vi "ReadForLoop.vi"(1 "reference":refnum<vi>) -> (0 "ForLoop":T6)   [LabVIEW 2013]
uses:
  <vilib>/Utility/miscctls.llb/LVBoundsTypeDef.ctl
  <vilib>/Utility/miscctls.llb/LVPositionTypeDef.ctl
  <vilib>/Utility/miscctls.llb/LVRectTypeDef.ctl
  <vilib>/Utility/miscctls.llb/LVBreakpointStatusEnum.ctl
  <vilib>/Utility/miscctls.llb/LVParallelSchedulesEnum.ctl
panel:
  out "error out 41":errorcluster
  out "error out 40":errorcluster
  out "error out 39":errorcluster
  out "error out 38":errorcluster
  out "error out 37":errorcluster
  out "error out 36":errorcluster
  out "error out 35":errorcluster
  out "error out 34":errorcluster
  out "error out 33":errorcluster
  out "error out 32":errorcluster
  out "error out 31":errorcluster
  out "error out 30":errorcluster
  out "error out 29":errorcluster
  out "error out 28":errorcluster
  out "error out 27":errorcluster
  out "error out 26":errorcluster
  out "error out 25":errorcluster
  out "error out 24":errorcluster
  out "error out 23":errorcluster
  out "error out 22":errorcluster
  out "error out 21":errorcluster
  out "error out 20":errorcluster
  out "error out 19":errorcluster
  out "error out 18":errorcluster
  out "error out 17":errorcluster
  out "error out 16":errorcluster
  out "error out 15":errorcluster
  out "error out 14":errorcluster
  out "error out 13":errorcluster
  out "error out 12":errorcluster
  out "error out 11":errorcluster
  out "error out 10":errorcluster
  out "error out 9":errorcluster
  out "error out 8":errorcluster
  out "error out 7":errorcluster
  out "error out 6":errorcluster
  out "error out 5":errorcluster
  out "error out 4":errorcluster
  out "error out 3":errorcluster
  out "error out 2":errorcluster
  out "error out":errorcluster
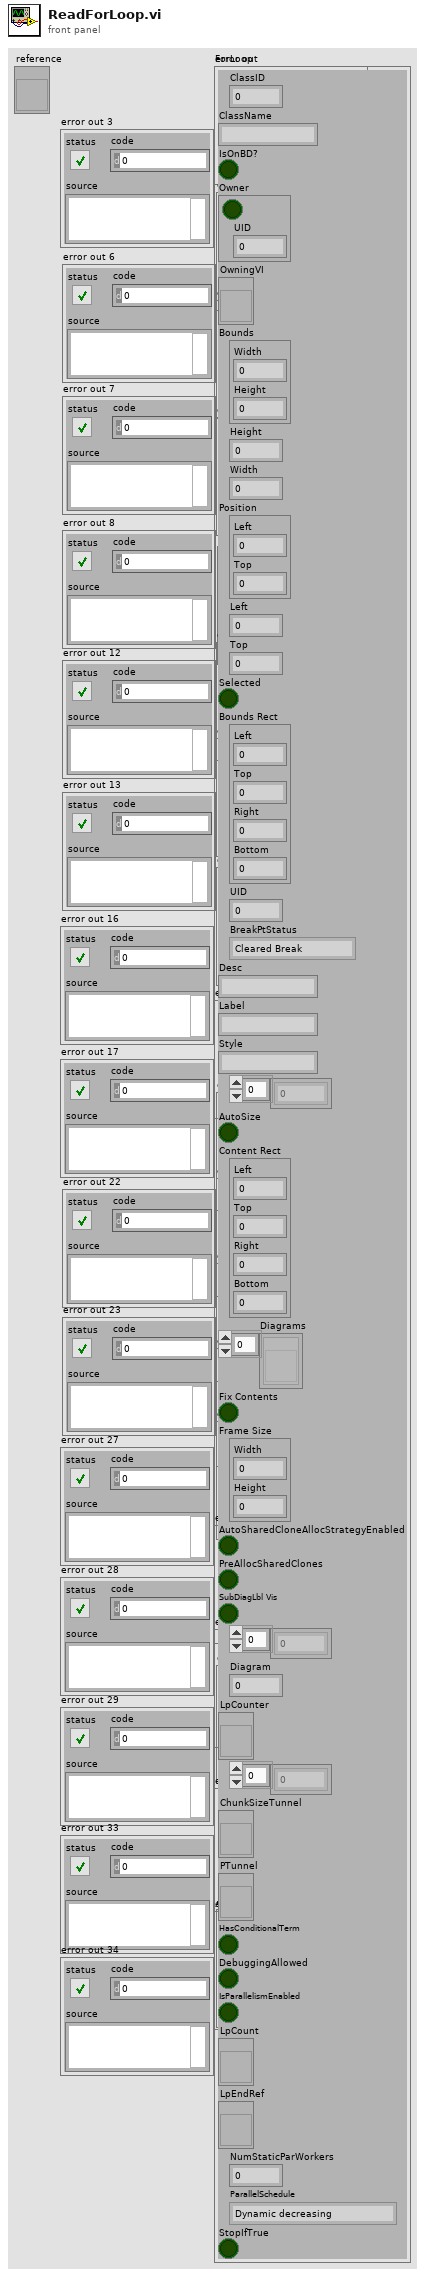
[diagram p1: front panel]
types:
  T1 = typedef "LVBoundsTypeDef.ctl" = cluster{"Width":u32, "Height":u32}
  T2 = typedef "LVPositionTypeDef.ctl" = cluster{"Left":i32, "Top":i32}
  T3 = typedef "LVRectTypeDef.ctl" = cluster{"Left":i16, "Top":i16, "Right":i16, "Bottom":i16}
  T4 = typedef "LVBreakpointStatusEnum.ctl" = enum8{"Cleared Break", "Enabled Break", "Disabled Break"}
  T5 = typedef "LVParallelSchedulesEnum.ctl" = enum8{"Dynamic decreasing", "Dynamic fixed size", "Static block", "Static block-cyclic"}
  T6 = cluster{"ClassID":u32, "ClassName":string, "IsOnBD?":bool, "Owner":cluster{bool, "UID":i32}, "OwningVI":refnum<vi>, "Bounds":T1, "Height":u32, "Width":u32, "Position":T2, "Left":i32, "Top":i32, "Selected":bool, "Bounds Rect":T3, "UID":i32, "BreakPtStatus":T4, "Desc":string, "Label":string, "Style":string, "Terms[]":i32[], "AutoSize":bool, "Content Rect":T3, "Diagrams":refnum<vi>[], "Fix Contents":bool, "Frame Size":T1, "AutoSharedCloneAllocStrategyEnabled":bool, "PreAllocSharedClones":bool, "SubDiagLbl Vis":bool, "Tunnels[]":i32[], "Diagram":i32, "LpCounter":refnum<vi>, "ShiftRegs[]":i32[], "ChunkSizeTunnel":refnum<vi>, "PTunnel":refnum<vi>, "HasConditionalTerm":bool, "DebuggingAllowed":bool, "IsParallelismEnabled":bool, "LpCount":refnum<vi>, "LpEndRef":refnum<vi>, "NumStaticParWorkers":i32, "ParallelSchedule":T5, "StopIfTrue":bool}
  T7 = cluster{"ClassID":u32, "ClassName":string, "IsOnBD?":bool, "Cluster":cluster{bool, "UID":i32}, "OwningVI":refnum<vi>, "Bounds":T1, "Height":u32, "Width":u32, "Position":T2, "Left":i32, "Top":i32, "Selected":bool, "Bounds Rect":T3, "UID":i32, "BreakPtStatus":T4, "Desc":string, "Text":string, "Style":string, i32[], "AutoSize":bool, "Content Rect":T3, "Diagrams":refnum<vi>[], "Fix Contents":bool, "Frame Size":T1, "AutoSharedCloneAllocStrategyEnabled":bool, "PreAllocSharedClones":bool, "SubDiagLbl Vis":bool, i32[], "UID":i32, "LpCounter":refnum<vi>, i32[], "ChunkSizeTunnel":refnum<vi>, "PTunnel":refnum<vi>, "HasConditionalTerm":bool, "DebuggingAllowed":bool, "IsParallelismEnabled":bool, "LpCount":refnum<vi>, "LpEndRef":refnum<vi>, "NumStaticParWorkers":i32, "ParallelSchedule":T5, "StopIfTrue":bool}
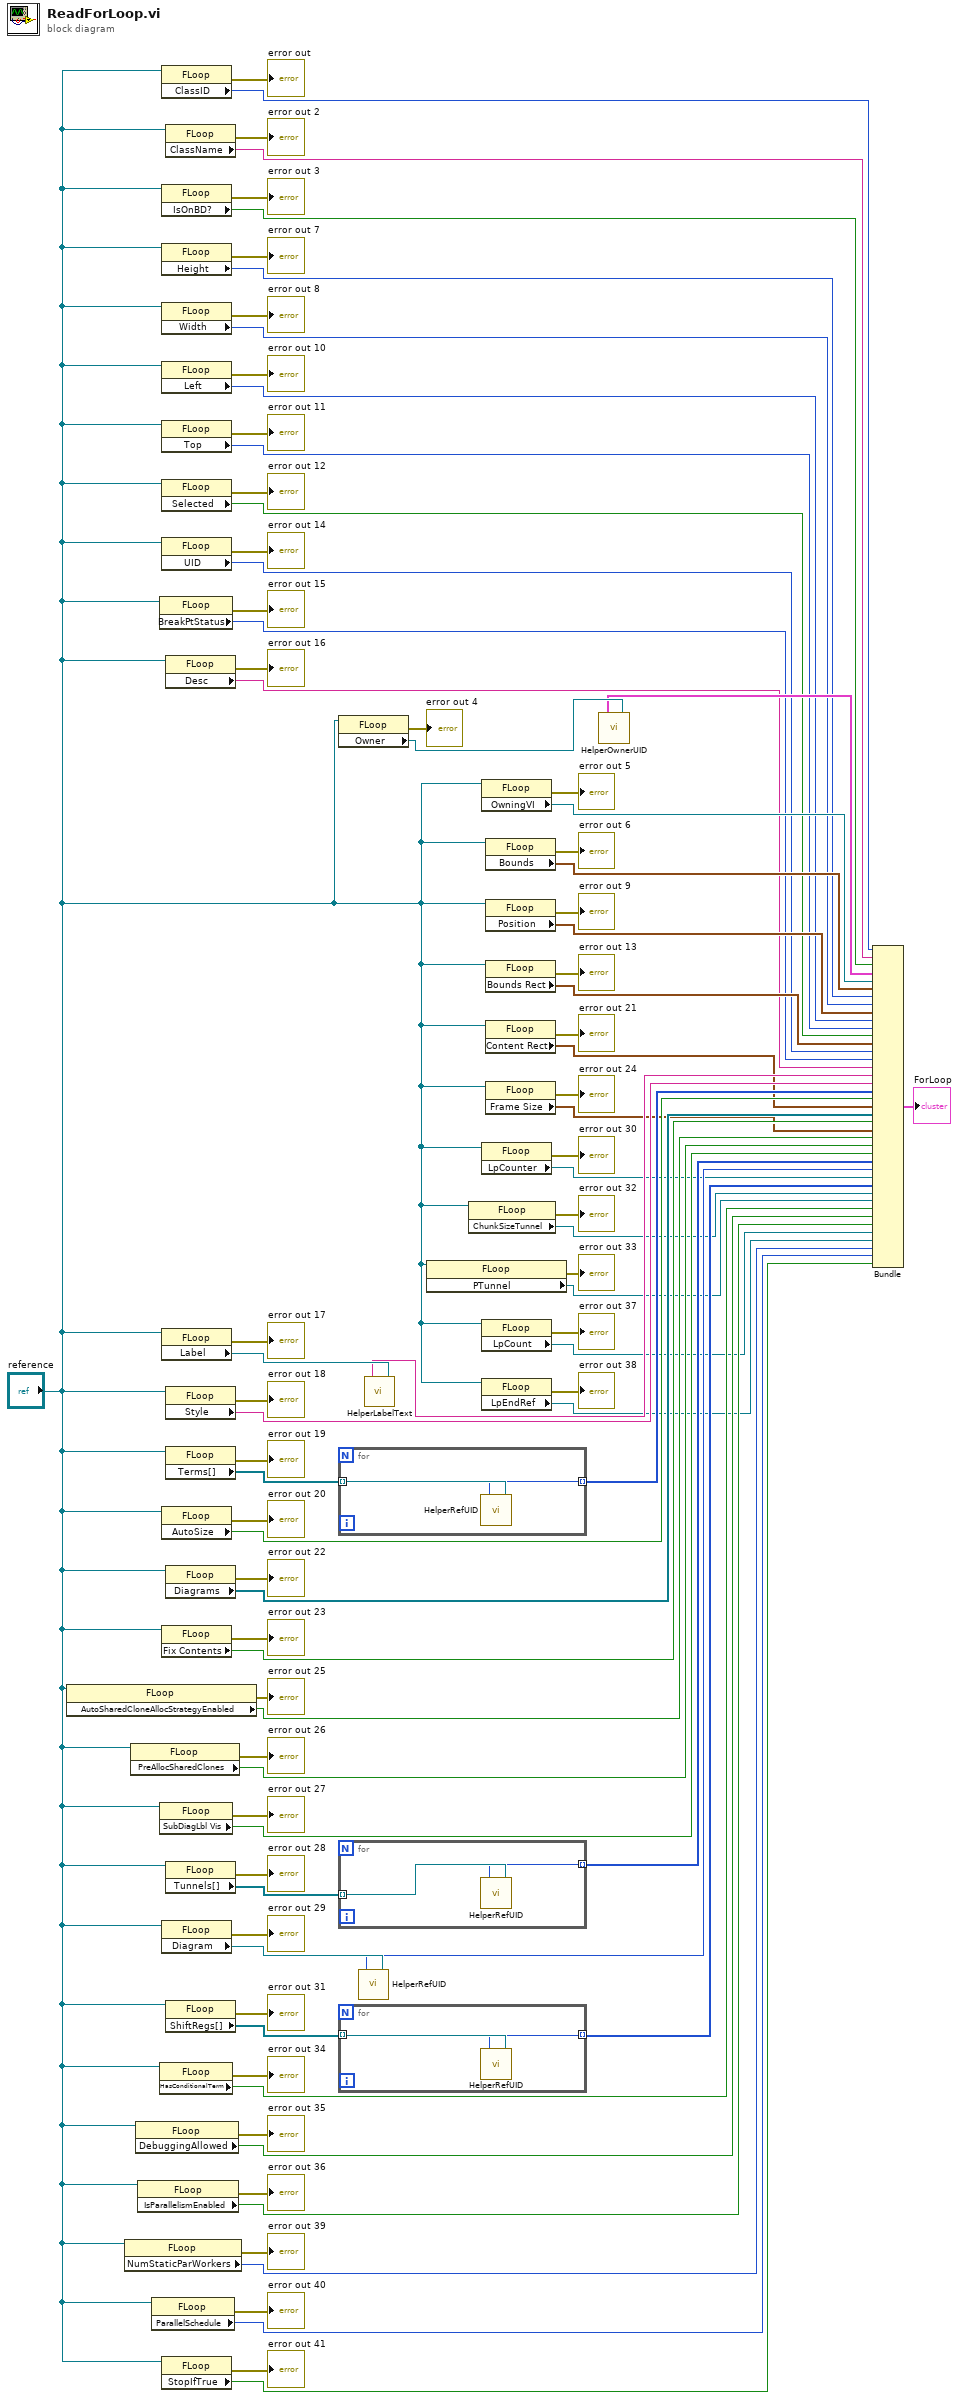
[diagram p0: block diagram]
diagram:
  n1 = property class="FLoop"(reference="reference") -> (error out=→"error out 25":errorcluster, "AutoSharedCloneAllocStrategyEnabled"=w37:bool)  [unwired: 1 in, 1 out]
  n2 = property class="FLoop"(reference="reference") -> (error out=→"error out 39":errorcluster, "NumStaticParWorkers"=w6:i32)  [unwired: 1 in, 1 out]
  n3 = property class="FLoop"(reference="reference") -> (error out=→"error out 26":errorcluster, "PreAllocSharedClones"=w35:bool)  [unwired: 1 in, 1 out]
  n4 = property class="FLoop"(reference="reference") -> (error out=→"error out 35":errorcluster, "DebuggingAllowed"=w14:bool)  [unwired: 1 in, 1 out]
  n5 = property class="FLoop"(reference="reference") -> (error out=→"error out 36":errorcluster, "IsParallelismEnabled"=w12:bool)  [unwired: 1 in, 1 out]
  n6 = property class="FLoop"(reference="reference") -> (error out=→"error out 40":errorcluster, "ParallelSchedule"=w4:T5)  [unwired: 1 in, 1 out]
  n7 = property class="FLoop"(reference="reference") -> (error out=→"error out 15":errorcluster, "BreakPtStatus"=w59:T4)  [unwired: 1 in, 1 out]
  n8 = property class="FLoop"(reference="reference") -> (error out=→"error out 27":errorcluster, "SubDiagLbl Vis"=w33:bool)  [unwired: 1 in, 1 out]
  n9 = property class="FLoop"(reference="reference") -> (error out=→"error out 34":errorcluster, "HasConditionalTerm"=w16:bool)  [unwired: 1 in, 1 out]
  n10 = property class="FLoop"(reference="reference") -> (error out=→"error out":errorcluster, "ClassID"=w88:u32)  [unwired: 1 in, 1 out]
  n11 = property class="FLoop"(reference="reference") -> (error out=→"error out 3":errorcluster, "IsOnBD?"=w84:bool)  [unwired: 1 in, 1 out]
  n12 = property class="FLoop"(reference="reference") -> (error out=→"error out 7":errorcluster, "Height"=w75:u32)  [unwired: 1 in, 1 out]
  n13 = property class="FLoop"(reference="reference") -> (error out=→"error out 8":errorcluster, "Width"=w73:u32)  [unwired: 1 in, 1 out]
  n14 = property class="FLoop"(reference="reference") -> (error out=→"error out 10":errorcluster, "Left"=w69:i32)  [unwired: 1 in, 1 out]
  n15 = property class="FLoop"(reference="reference") -> (error out=→"error out 11":errorcluster, "Top"=w67:i32)  [unwired: 1 in, 1 out]
  n16 = property class="FLoop"(reference="reference") -> (error out=→"error out 12":errorcluster, "Selected"=w65:bool)  [unwired: 1 in, 1 out]
  n17 = property class="FLoop"(reference="reference") -> (error out=→"error out 14":errorcluster, "UID"=w61:i32)  [unwired: 1 in, 1 out]
  n18 = property class="FLoop"(reference="reference") -> (error out=→"error out 17":errorcluster, "Label"=w55:refnum<vi>)  [unwired: 1 in, 1 out]
  n19 = property class="FLoop"(reference="reference") -> (error out=→"error out 20":errorcluster, "AutoSize"=w47:bool)  [unwired: 1 in, 1 out]
  n20 = property class="FLoop"(reference="reference") -> (error out=→"error out 23":errorcluster, "Fix Contents"=w41:bool)  [unwired: 1 in, 1 out]
  n21 = property class="FLoop"(reference="reference") -> (error out=→"error out 29":errorcluster, "Diagram"=w28:refnum<vi>)  [unwired: 1 in, 1 out]
  n22 = property class="FLoop"(reference="reference") -> (error out=→"error out 41":errorcluster, "StopIfTrue"=w2:bool)  [unwired: 1 in, 1 out]
  n23 = property class="FLoop"(reference="reference") -> (error out=→"error out 2":errorcluster, "ClassName"=w86:string)  [unwired: 1 in, 1 out]
  n24 = property class="FLoop"(reference="reference") -> (error out=→"error out 16":errorcluster, "Desc"=w57:string)  [unwired: 1 in, 1 out]
  n25 = property class="FLoop"(reference="reference") -> (error out=→"error out 18":errorcluster, "Style"=w52:string)  [unwired: 1 in, 1 out]
  n26 = property class="FLoop"(reference="reference") -> (error out=→"error out 19":errorcluster, "Terms[]"=w50:refnum<vi>[])  [unwired: 1 in, 1 out]
  n27 = property class="FLoop"(reference="reference") -> (error out=→"error out 22":errorcluster, "Diagrams"=w43:refnum<vi>[])  [unwired: 1 in, 1 out]
  n28 = property class="FLoop"(reference="reference") -> (error out=→"error out 28":errorcluster, "Tunnels[]"=w31:refnum<vi>[])  [unwired: 1 in, 1 out]
  n29 = property class="FLoop"(reference="reference") -> (error out=→"error out 31":errorcluster, "ShiftRegs[]"=w23:refnum<vi>[])  [unwired: 1 in, 1 out]
  n30 = property class="FLoop"(reference="reference") -> (error out=→"error out 4":errorcluster, "Owner"=w82:refnum<vi>)  [unwired: 1 in, 1 out]
  n31 = for {
    tunnel: w50 -> [w92] mode=indexing
    tunnel: [w91] -> w49 mode=indexing
    n32 = call "HelperRefUID.vi"("Text in"=w92) -> ("UID"=w91:i32)
  }
  n33 = for {
    tunnel: w31 -> [w94] mode=indexing
    tunnel: [w93] -> w30 mode=indexing
    n34 = call "HelperRefUID.vi"("Text in"=w94) -> ("UID"=w93:i32)
  }
  n35 = for {
    tunnel: w23 -> [w96] mode=indexing
    tunnel: [w95] -> w22 mode=indexing
    n36 = call "HelperRefUID.vi"("Text in"=w96) -> ("UID"=w95:i32)
  }
  n37 = call "HelperRefUID.vi"("Text in"=w28) -> ("UID"=w27:i32)
  n38 = call "HelperLabelText.vi"("Text in"=w55) -> ("Text"=w54:string)
  n39 = property class="FLoop"(reference="reference") -> (error out=→"error out 33":errorcluster, "PTunnel"=w18:refnum<vi>)  [unwired: 1 in, 1 out]
  n40 = property class="FLoop"(reference="reference") -> (error out=→"error out 32":errorcluster, "ChunkSizeTunnel"=w20:refnum<vi>)  [unwired: 1 in, 1 out]
  n41 = property class="FLoop"(reference="reference") -> (error out=→"error out 5":errorcluster, "OwningVI"=w79:refnum<vi>)  [unwired: 1 in, 1 out]
  n42 = property class="FLoop"(reference="reference") -> (error out=→"error out 30":errorcluster, "LpCounter"=w25:refnum<vi>)  [unwired: 1 in, 1 out]
  n43 = property class="FLoop"(reference="reference") -> (error out=→"error out 37":errorcluster, "LpCount"=w10:refnum<vi>)  [unwired: 1 in, 1 out]
  n44 = property class="FLoop"(reference="reference") -> (error out=→"error out 38":errorcluster, "LpEndRef"=w8:refnum<vi>)  [unwired: 1 in, 1 out]
  n45 = property class="FLoop"(reference="reference") -> (error out=→"error out 6":errorcluster, "Bounds"=w77:T1)  [unwired: 1 in, 1 out]
  n46 = property class="FLoop"(reference="reference") -> (error out=→"error out 9":errorcluster, "Position"=w71:T2)  [unwired: 1 in, 1 out]
  n47 = property class="FLoop"(reference="reference") -> (error out=→"error out 13":errorcluster, "Bounds Rect"=w63:T3)  [unwired: 1 in, 1 out]
  n48 = property class="FLoop"(reference="reference") -> (error out=→"error out 21":errorcluster, "Content Rect"=w45:T3)  [unwired: 1 in, 1 out]
  n49 = property class="FLoop"(reference="reference") -> (error out=→"error out 24":errorcluster, "Frame Size"=w39:T1)  [unwired: 1 in, 1 out]
  n50 = call "HelperOwnerUID.vi"("Generic in"=w82) -> ("Cluster"=w81:cluster{bool, "UID":i32})
  n51 = Bundle("ClassID"=w88, "ClassName"=w86, "IsOnBD?"=w84, "Cluster"=w81, "OwningVI"=w79, "Bounds"=w77, "Height"=w75, "Width"=w73, "Position"=w71, "Left"=w69, "Top"=w67, "Selected"=w65, "Bounds Rect"=w63, "UID"=w61, "BreakPtStatus"=w59, "Desc"=w57, "Text"=w54, "Style"=w52, w49, "AutoSize"=w47, "Content Rect"=w45, "Diagrams"=w43, "Fix Contents"=w41, "Frame Size"=w39, "AutoSharedCloneAllocStrategyEnabled"=w37, "PreAllocSharedClones"=w35, "SubDiagLbl Vis"=w33, w30, "UID"=w27, "LpCounter"=w25, w22, "ChunkSizeTunnel"=w20, "PTunnel"=w18, "HasConditionalTerm"=w16, "DebuggingAllowed"=w14, "IsParallelismEnabled"=w12, "LpCount"=w10, "LpEndRef"=w8, "NumStaticParWorkers"=w6, "ParallelSchedule"=w4, "StopIfTrue"=w2) -> (→"ForLoop":T7)  [unwired: 1 in]
